vi "test Set and Get Properties.vi"(8 "error in (no error)":errorcluster, 11 "TestCase in":refnum<class "SLSC Switch Scripting Unit Tests.lvclass">) -> (0 "error out":errorcluster, 3 "TestCase out":refnum<class "SLSC Switch Scripting Unit Tests.lvclass">)   [LabVIEW 2017, in "SLSC Switch Scripting Unit Tests.lvclass"]
uses:
  SLSC Switch Scripting Unit Tests.lvclass
  Properties/SLSC Switch All Properties.ctl
  SLSC Switch Scripting Unit Tests.lvclass/SLSC Switch Scripting Unit Tests.ctl
  <vilib>/addons/_JKI Toolkits/VI Tester/TestCase.llb/TestCase.lvclass
  SLSC Switch Scripting.lvlib
  C:/Program Files (x86)/National Instruments/LabVIEW 2017/vi.lib/addons/_JKI Toolkits/VI Tester/TestCase.llb/TestCase.lvclass
panel:
  in  "Save?":bool
  out "Output Filename":string
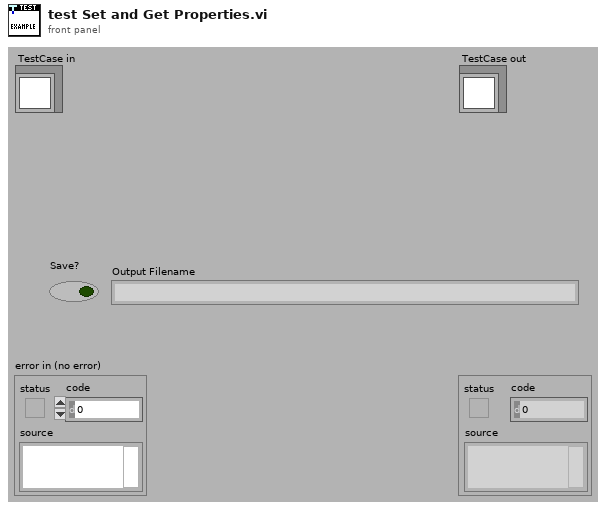
[diagram p1: front panel]
types:
  T1 = typedef "SLSC Switch Scripting.lvlib/SLSC Switch All Properties.ctl" = cluster{"Model":string, "Resource":string, "Topology":string, "Capabilities":string}
  T2 = typedef "Custom Device API.lvlib/Custom Device Item Ref.ctl" = u64
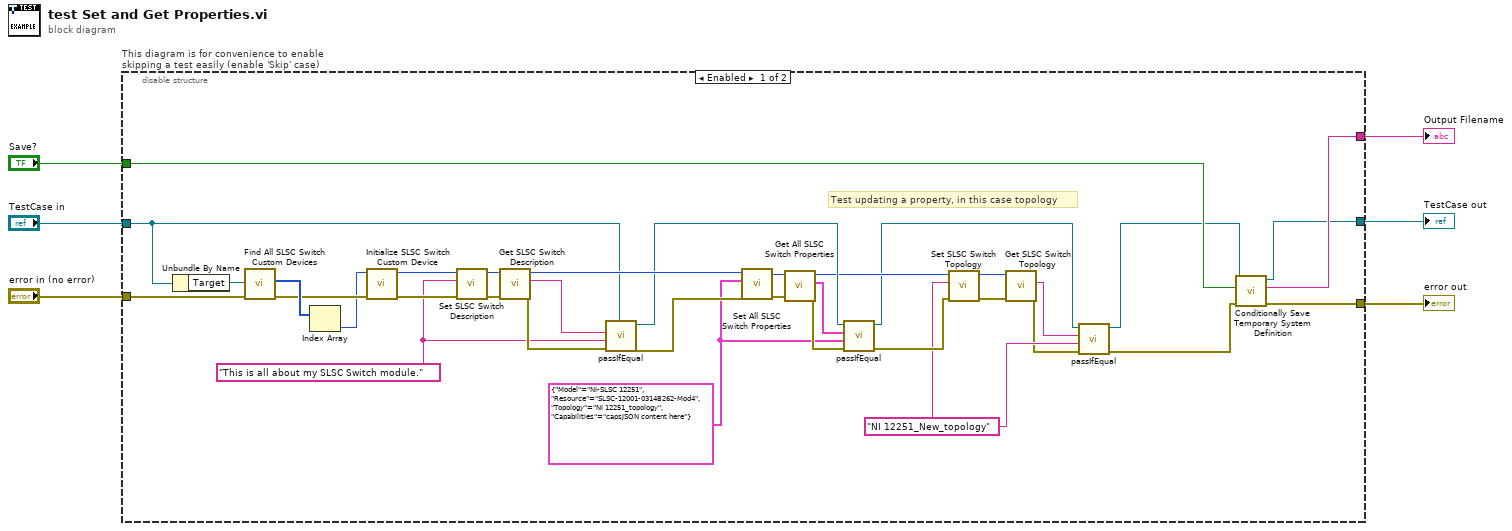
[diagram p0: block diagram]
diagram:
  n1 = disable-structure "This diagram is for convenience to enable skipping a test easily (enable 'Skip' case)" shown="Enabled" {
    disable-tunnel: "TestCase in" -> [w27 w45]
    disable-tunnel: [w39 w43] -> w3
    disable-tunnel: [w40 w44] -> w5
    disable-tunnel: "error in (no error)" -> [w33 w42]
    disable-tunnel: [w41 _] -> w2
    disable-tunnel: "Save?" -> [w38 _]
    frame Enabled {
      w7 = T1 {"Model"="NI-SLSC 12251", "Resource"="SLSC-12001-0314B262-Mod4", "Topology"="NI 12251_topology", "Capabilities"="capsJSON content here"} ("SLSC Switch All Properties")
      w12 = "NI 12251_New_topology" ("Topology")
      w22 = "This is all about my SLSC Switch module." ("Description")
      # "Test updating a property, in this case topology"
      n2 = Unbundle By Name(w27) -> ("Target"=w34:refnum<k24>)
      n3 = call "Find All SLSC Switch Custom Devices.vi"("error in (no error)"=w33, "Target in"=w34) -> ("error out"=w36:errorcluster, "SLSC Switch Custom Device Ref IDs"=w37:T2[])  [unwired: 7 in, 1 out]
      n4 = Index Array(array=w37) -> (element=w35:T2)  [unwired: 1 in]
      n5 = call "Initialize SLSC Switch Custom Device.vi"("error in (no error)"=w36, "SLSC Switch Custom Device Ref in"=w35) -> ("error out"=w31:errorcluster, "SLSC Switch Custom Device Ref out"=w32:T2)  [unwired: 7 in, 1 out]
      n6 = call "Set SLSC Switch Description.vi"("error in (no error)"=w31, "Description"=w22, "SLSC Switch Custom Device Ref in"=w32) -> ("error out"=w24:errorcluster, "SLSC Switch Custom Device Ref out"=w30:T2)  [unwired: 7 in]
      n7 = call "Get SLSC Switch Description.vi"("error in (no error)"=w24, "SLSC Switch Custom Device Ref in"=w30) -> ("error out"=w25:errorcluster, "Description"=w28:string, "SLSC Switch Custom Device Ref out"=w29:T2)  [unwired: 7 in]
      n8 = call-dynamic "passIfEqual.vi"("error in (no error)"=w25, "y"=w22, "x"=w28, "TestCase in"=w27) -> ("error out"=w23:errorcluster, "TestCase out"=w26:refnum<class "SLSC Switch Scripting Unit Tests.lvclass">)  [unwired: 6 in]
      n9 = call "Set All SLSC Switch Properties.vi"("error in (no error)"=w23, "SLSC Switch All Properties"=w7, "SLSC Switch Custom Device Ref in"=w29) -> ("error out"=w18:errorcluster, "SLSC Switch Custom Device Ref out"=w19:T2)  [unwired: 7 in]
      n10 = call "Get All SLSC Switch Properties.vi"("error in (no error)"=w18, "SLSC Switch Custom Device Ref in"=w19) -> ("error out"=w21:errorcluster, "SLSC Switch All Properties"=w20:T1, "SLSC Switch Custom Device Ref out"=w17:T2)  [unwired: 7 in]
      n11 = call-dynamic "passIfEqual.vi"("error in (no error)"=w21, "y"=w7, "x"=w20, "TestCase in"=w26) -> ("error out"=w16:errorcluster, "TestCase out"=w10:refnum<class "SLSC Switch Scripting Unit Tests.lvclass">)  [unwired: 6 in]
      n12 = call "Set SLSC Switch Topology.vi"("error in (no error)"=w16, "Topology"=w12, "SLSC Switch Custom Device Ref in"=w17) -> ("error out"=w14:errorcluster, "SLSC Switch Custom Device Ref out"=w15:T2)  [unwired: 7 in]
      n13 = call "Get SLSC Switch Topology.vi"("error in (no error)"=w14, "SLSC Switch Custom Device Ref in"=w15) -> ("error out"=w11:errorcluster, "Topology"=w13:string)  [unwired: 7 in, 1 out]
      n14 = call-dynamic "passIfEqual.vi"("error in (no error)"=w11, "y"=w12, "x"=w13, "TestCase in"=w10) -> ("error out"=w8:errorcluster, "TestCase out"=w9:refnum<class "SLSC Switch Scripting Unit Tests.lvclass">)  [unwired: 6 in]
      n15 = call "Conditionally Save Temporary System Definition.vi"("error in (no error)"=w8, "Save?"=w38, "Test Case"=w9) -> ("error out"=w40:errorcluster, "filename"=w41:string, "Test Case"=w39:refnum<class "SLSC Switch Scripting Unit Tests.lvclass">)  [unwired: 6 in]
    }
    frame Disabled {
      # "skip test result while test is under development"
      n16 = call <vilib>:"skip.vi"("error in (no error)"=w42, "TestCase in"=w45) -> ("error out"=w44:errorcluster, "TestCase out"=w43:refnum<class "SLSC Switch Scripting Unit Tests.lvclass">)  [unwired: 8 in]
    }
  }
  "error out" <- w5
  "TestCase out" <- w3
  "Output Filename" <- w2
